vi "Generate Error.vi"(5 "<err> (\"\")":string, 7 "<append> (\"\")":string, 8 "error in (no error)":errorcluster, 10 "chain levels to remove (1)":i32=1 min=1, 11 "code":i32) -> (0 "error out":errorcluster)   [LabVIEW 2017, in "NI_Robotics Utilities.lvlib"]
uses:
  <vilib>/robotics/Utilities/NI_Robotics Utilities.lvlib
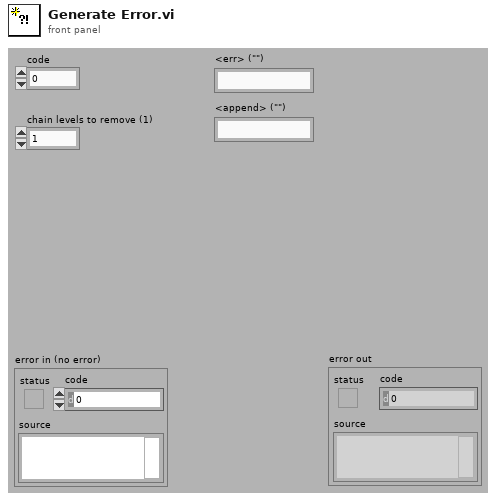
[diagram p1: front panel]
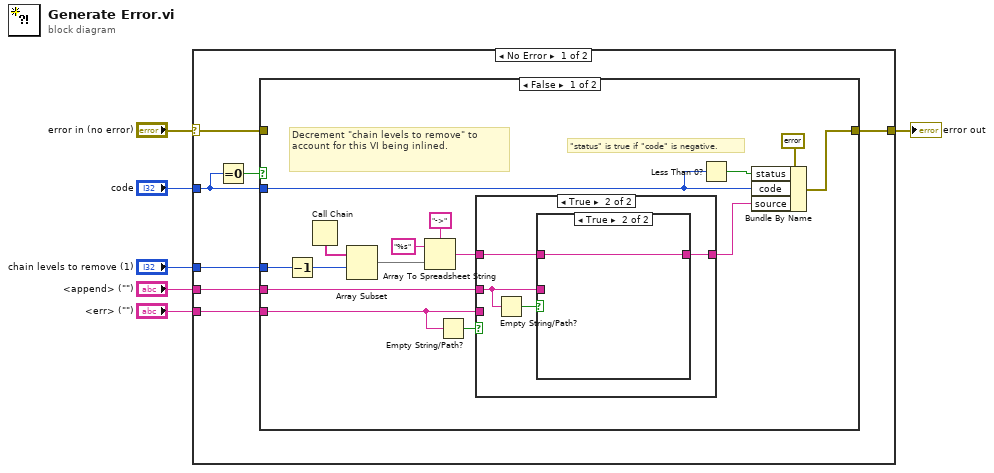
[diagram p0: block diagram]
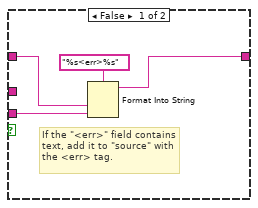
[diagram p2: hidden frame]
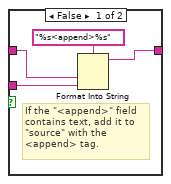
[diagram p3: hidden frame]
diagram:
  n1 = case shown="No Error" "error in (no error)" {
    selector: "error in (no error)" -> [w11 w43]
    tunnel: [w12 w43] -> w5
    tunnel: "code" -> [w10 _]
    tunnel: "chain levels to remove (1)" -> [w13 _]
    tunnel: "<err> (\"\")" -> [w9 _]
    tunnel: "<append> (\"\")" -> [w8 _]
    frame No Error {
      n2 = Equal To 0?(x=w10) -> (x = 0?=w7:bool)
      n3 = case shown="False" w7 {
        tunnel: w11 -> [_ w42]
        tunnel: w13 -> [w27 _]
        tunnel: [w25 w42] -> w12
        tunnel: w10 -> [w21 _]
        tunnel: w9 -> [w18 _]
        tunnel: w8 -> [w17 _]
        frame False {
          # "Decrement \"chain levels to remove\" to account for this VI being inlined."
          # "\"status\" is true if \"code\" is negative."
          n4 = Decrement(x=w27) -> (x-1=w14:i32)
          n5 = Call Chain() -> (call chain=w28:string[])
          n6 = Array Subset(array=w28, index=w14) -> (w24:string[])  [unwired: 1 in]
          n7 = Array To Spreadsheet String(delimiter (Tab)="->", array=w24, 3:"%s" ("format string")) -> (spreadsheet string=w20:string)
          n8 = Empty String/Path?(string/path=w18) -> (empty?=w19:bool)
          n9 = case shown="True" w19 {
            tunnel: w20 -> [w29 w34]
            tunnel: w18 -> [w30 _]
            tunnel: w17 -> [_ w35]
            tunnel: [w31 w33] -> w16
            frame False {
              # "If the \"<err>\" field contains text, add it to \"source\" with the <err> tag."
              n10 = Format Into String(format string="%s<err>%s", w29, w30) -> (resulting string=w31:string)  [unwired: 2 in, 1 out]
            }
            frame True {
              n11 = Empty String/Path?(string/path=w35) -> (empty?=w36:bool)
              n12 = case shown="True" w36 {
                tunnel: w35 -> [w39 _]
                tunnel: w34 -> [w40 w41]
                tunnel: [w37 w41] -> w33
                frame False {
                  # "If the \"<append>\" field contains text, add it to \"source\" with the <append> tag."
                  n13 = Format Into String(format string="%s<append>%s", w40, w39) -> (resulting string=w37:string)  [unwired: 2 in, 1 out]
                }
                frame True {
                }
              }
            }
          }
          n14 = Less Than 0?(x=w21) -> (x < 0?=w26:bool)
          n15 = Bundle By Name(cluster=errorcluster {"status"=FALSE, "code"=0, "source"=""} ("error IO"), "status"=w26, "code"=w21, "source"=w16) -> (w25:errorcluster)
        }
        frame True {
          # "Do nothing if the new code is zero."
        }
      }
    }
    frame Error {
      # "Do nothing if there is already an error on the wire."
    }
  }
  "error out" <- w5
